vi "Read MainWindowPosition.vi"(8 "error in (no error)":errorcluster, 11 "Preferences in":refnum<class "SetListPrefs.lvclass">) -> (0 "error out":errorcluster, 2 "MainWindowPosition":T2, 3 "Preferences out":refnum<class "SetListPrefs.lvclass">)   [LabVIEW 2013, in "SetListPrefs.lvclass"]
uses:
  SetListPrefs.lvclass
  <vilib>/Utility/miscctls.llb/LVRectTypeDef.ctl
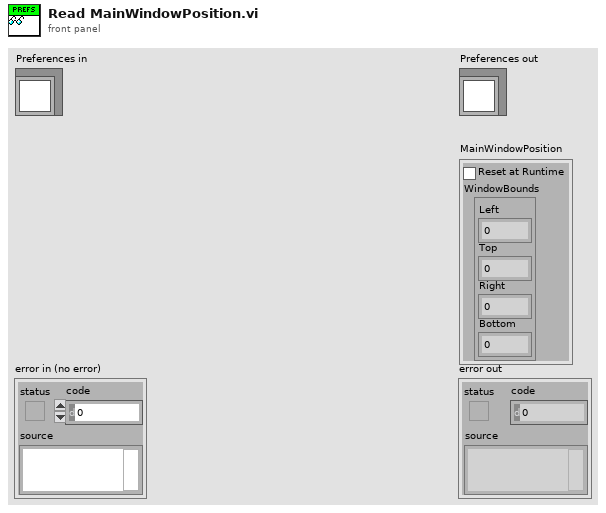
[diagram p1: front panel]
types:
  T1 = typedef "LVRectTypeDef.ctl" = cluster{"Left":i16, "Top":i16, "Right":i16, "Bottom":i16}
  T2 = cluster{"Reset at Runtime":bool, "WindowBounds":T1}
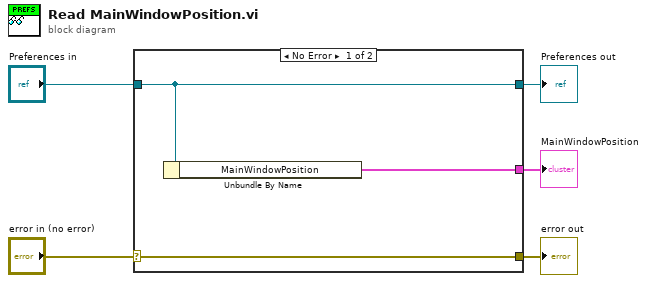
[diagram p0: block diagram]
diagram:
  n1 = case shown="No Error" "error in (no error)" {
    selector: "error in (no error)" -> [w8 w9]
    tunnel: [w8 w9] -> w4
    tunnel: [w7 w10] -> w2
    tunnel: "Preferences in" -> [w7 w10]
    tunnel: [w6 _] -> w1
    frame No Error {
      n2 = Unbundle By Name(w7) -> ("MainWindowPosition"=w6:T2)
    }
    frame Error {
    }
  }
  "error out" <- w4
  "Preferences out" <- w2
  "MainWindowPosition" <- w1
